vi "Scan Engine-Single Frame.vi"(8 "Error in":errorcluster, 10 "Scan Status":enum16{"Start", "Continue Scan", "Finish Scan"}(ring)=enum."Continue Scan", 11 "Scan Type in":T1) -> (0 "Error Out":errorcluster, 3 "data out":sgl[](array[numeric]))   [LabVIEW 2018]
uses:
  Controls/ScanType.ctl
  Hardware Mfg/AlazarTech SDK/Controls/Alazar Engine Actions.ctl
  Controls/Queue Manager Actions.ctl
  Controls/FGV Actions.ctl
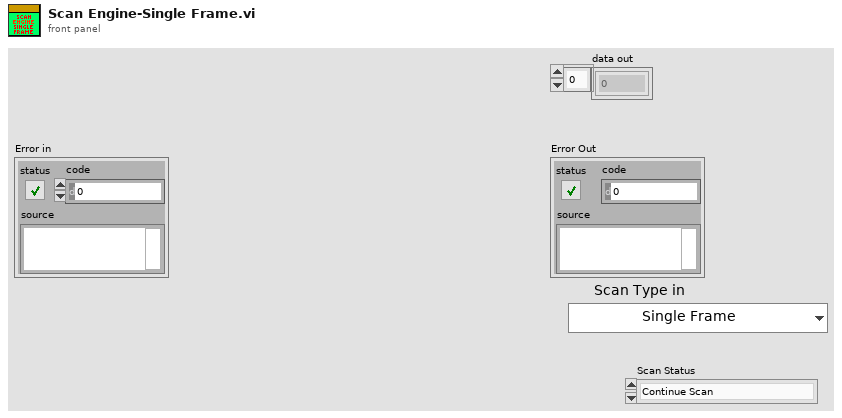
[diagram p1: front panel]
types:
  T1 = typedef "ScanType.ctl" = enum16{"Single Frame", "Continuous Frame", "ROI Line", "Vibratome", "Mosaic", "Mosaic + Slice"}
  T2 = typedef "FGV Actions.ctl" = enum16{"Init", "Set", "Get", "Clear"}
  T3 = typedef "Alazar Engine Actions.ctl" = enum16{"Init", "Config Clock", "Config Ch", "Config Trig", "Config Non-FFT Acq.", "Non-FFT Acquire", "Load background from Non-FFT buffer", "enable background subtrac", "disable background subtrac", "load background from file", "load background from elsewhere", "start acquire", "background subtraction", "Config Acq.", "Acquire", "UnInit"}
  T4 = enum16{"Configure channels", "Write Scan Pattern", "Start Galvo Task", "Is Task Done?", "Stop Galvo", "Uninit", "Init: Calc scan pattern"}
  T5 = typedef "Queue Manager Actions.ctl" = enum16{"Init", "Enqueue", "Enqueue All", "Preview Queue", "Dequeue", "Get Status", "Flush Queue", "Flush All Queues", "Release All Queues", "Release Queue", "Enqueue at Opposite End"}
  T6 = typedef "Alazar parameters.ctl" = cluster{"Trigger Settings":cluster{"General Trigger Settings":T7, "Trigger Engine 1":T8, "Trigger Engine 2":T8}, "Capture Clock":T9, "Device ID":T10, "Ch A Input Control":T11, "Ch B Input Control":T11, "Acq Settings":T12, "Cluster":T13}
  T7 = typedef "General Trigger Settings.ctl" = cluster{"Trigger Operation":u32, "Coupling ID":u32, "Range ID":u32, "Delay":u32, "Timeout Ticks":u32, "Mode":u32, "Parameter":u32}
  T8 = typedef "Trigger Engine Controls.ctl" = cluster{"Trigger Engine":u32, "Source":u32, "Slope":u32, "Level":u32}
  T9 = typedef "Clock Controls.ctl" = cluster{"Sample Rate":u32, "Decimation":u32, "Source":u32, "Edge":u32}
  T10 = typedef "Alazar Device ID.ctl" = cluster{"System ID":u32, "Board ID":u32}
  T11 = typedef "Channel Input Controls.ctl" = cluster{"Channel":u8, "Coupling":u32, "Range":u32, "Impedance":u32}
  T12 = typedef "Alazar Acquisition Settings.ctl" = cluster{"Window Type":u32, "Record Length":u32, "Footer":u32, "Output Format":u32, "Offset":u32, "Records Per Buffer":u32, "Samples per record":u32, "Records Count (Records/Acq)":u32}
  T13 = typedef "Control cluster.ctl" = cluster{"FFT value magnification":dbl, "max queue size (-1, unlimited)":i32, "File Type":T14, "file path":path, "#A-lines to save":u32, "#Z pixels to save":u32, "ImageDescription":string, "Convert to U16?":bool}
  T14 = typedef "file type.ctl" = enum16{"text", "Tiff", "binary"}
  T15 = cluster{"General Trigger Settings":T7, "Trigger Engine 1":T8, "Trigger Engine 2":T8}
  T16 = typedef "Galvo parameters.ctl" = cluster{"Galvo HW Parameters":cluster{"Analog Out Channel":tag, "Min Voltage":dbl, "Max Voltage":dbl, "Pixel Clock Source":tag, "Sample Rate":dbl, "Line Clock Out Ch":tag}, "System Parameters":T17}
  T17 = typedef "System Parameters.ctl" = cluster{"Optical Parameters":T18, "Vibratome":T19, "Table Stages":T20, "Imaging Parameter":T23}
  T18 = typedef "Optical Parameters.ctl" = cluster{"Obj. Focal Length [mm]":dbl, "Scan Lens EFL[mm]":dbl, "Tube Lens EFL[mm]":dbl, "Galvo V Range (+/-)":dbl, "Galvo Max Half Angle [Deg]":dbl, "Max Galvo Range[%]":dbl}
  T19 = typedef "Vibratome Parameters.ctl" = cluster{"Z Bottom [mm]":dbl, "Pre Cut Dwell [s]":dbl, "Blade Frequency [RPM]":u16, "Slice Speed [mm/s]":dbl, "Post Cut Dwell [s]":dbl, "Ramp Time [s]":dbl, "Start X [mm]":dbl, "Start Y [mm]":dbl, "Slice Length [mm]":dbl, "Slice Axis":enum16{"X Axis", "Y Axis", "Z Axis"}, "Controller VISA Ref":refnum<visa-resource-name>}
  T20 = typedef "Translation Stage Parameters.ctl" = cluster{"X Stage":T21, "Y Stage":T21, "Z Stage":T21}
  T21 = typedef "Translation Stage Cluster.ctl" = cluster{"Position":dbl, "Is.Enabled?":bool, "Is.Connected?":bool, "Device SN":string, "AccelerationMaximum":dbl, "VelocityMaximum":dbl, "Acceleration":dbl, "Velocity":dbl, "waitTimeout (ms)":i32, "Model":T22, "Is.Homed?":bool}
  T22 = typedef "Translation Stage Types.ctl" = enum16{"None", "Thorlabs LTS", "Thorlabs MLJ"}
  T23 = typedef "Imaging Parameters.ctl" = cluster{"Raster Scan Direction":T24, "Pixel Dwell Time [Clock Cycles]":u16, "Flyback Time [Clock Cycles]":u16, "XY Center [um]":cluster{"X":dbl, "Y":dbl}, "Pixel Step Size [um]":dbl, "XY Image Size":enum16{"32 x 32", "64 x 64", "128 x 128", "256 x 256", "512 x 512", "1024 x 1024", "2048 x 2048"}, "Custom":bool, "Custom Size":cluster{"X":u16, "Y":u16}, "Line Averages":u8}
  T24 = typedef "Scan Direction.ctl" = enum16{"Uni Directional", "Bi Directional", "None"}
  T25 = cluster{"Analog Out Channel":tag, "Min Voltage":dbl, "Max Voltage":dbl, "Pixel Clock Source":tag, "Sample Rate":dbl, "Line Clock Out Ch":tag}
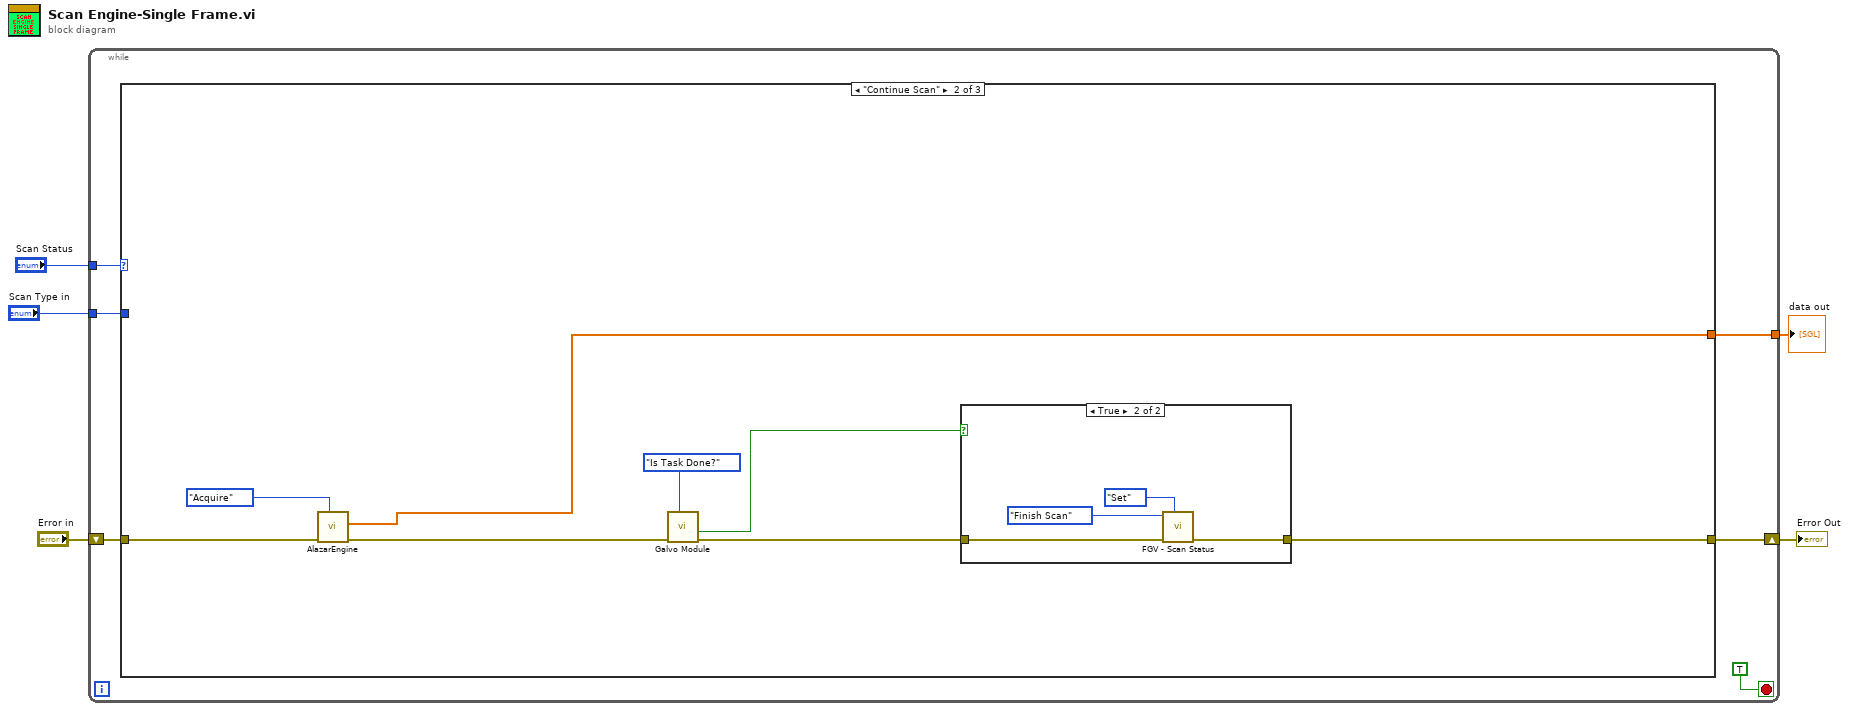
[diagram p0: block diagram]
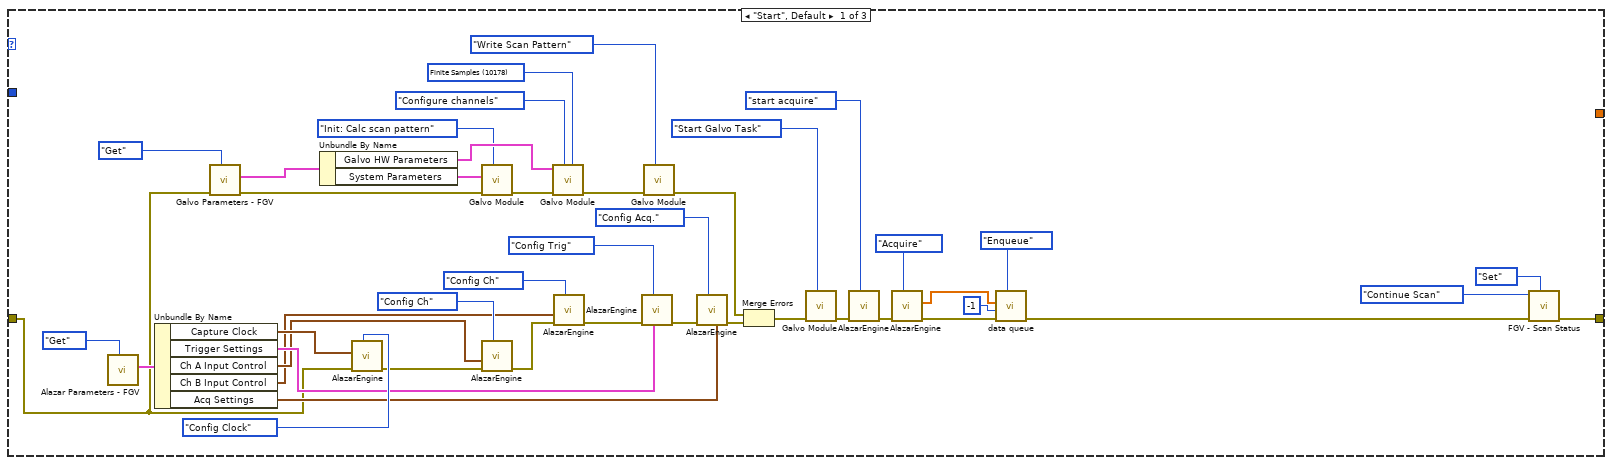
[diagram p2: hidden frame]
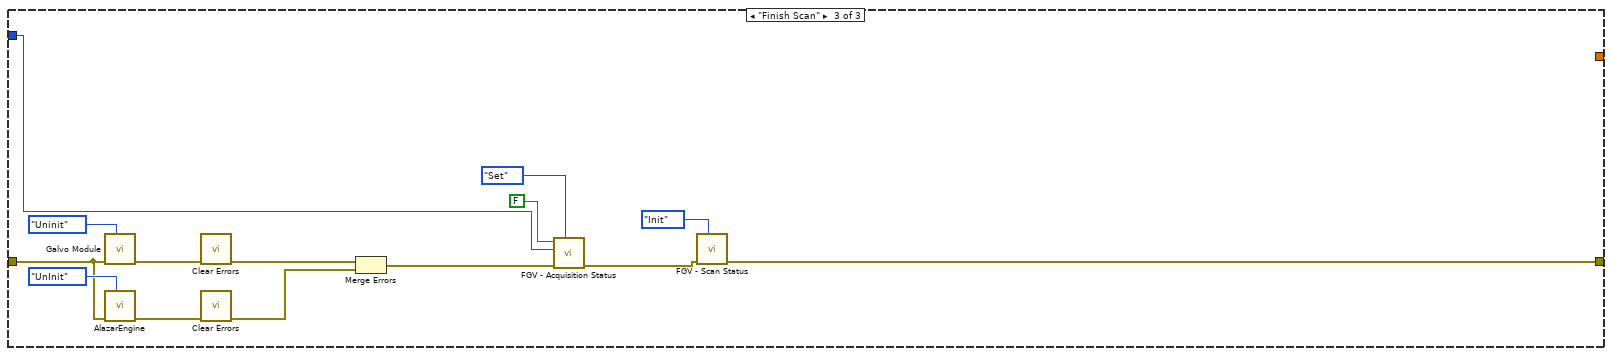
[diagram p4: hidden frame]
diagram:
  n1 = while {
    shift-right: [w10] -> w4
    shift-left: "Error in" -> [w7]
    tunnel: "Scan Type in" -> [w9]
    tunnel: "Scan Status" -> [w8]
    tunnel: [w6] -> w1
    stop <- TRUE ("Status In") stop-if-true
    n2 = case shown="\"Continue Scan\"" w8 {
      tunnel: w7 -> [w16 w61 w78]
      tunnel: [w15 w60 w69] -> w10
      tunnel: w9 -> [_ _ w72]
      tunnel: [_ w56 _] -> w6
      frame "Start", Default {
        w42 = 10178 items=["Finite Samples"=10178, "Continuous Samples"=10123, "Hardware Timed Single Point"=12522] ("sample mode")
        n3 = call "Alazar Parameters - FGV.vi"("Actions"=FGV_Actions."Get") -> ("Alazar parameters out"=w28:T6)  [unwired: 9 in, 1 out]
        n4 = Unbundle By Name(w28) -> ("Capture Clock"=w27:T9, "Trigger Settings"=w26:T15, "Ch A Input Control"=w25:T11, "Ch B Input Control"=w24:T11, "Acq Settings"=w23:T12)
        n5 = call "Galvo Parameters - FGV.vi"("Actions"=FGV_Actions."Get", "Error In"=w16) -> ("Error Out"=w49:errorcluster, "Galvo parameters out"=w44:T16)  [unwired: 8 in]
        n6 = Unbundle By Name(w44) -> ("Galvo HW Parameters"=w47:T25, "System Parameters"=w48:T17)
        n7 = call "AlazarEngine.vi"("Action"=Alazar_Engine_Actions."Config Clock", "error in (no error)"=w16, "Capture Clock"=w27) -> ("error out"=w31:errorcluster)  [unwired: 7 in, 1 out]
        n8 = call "Galvo Module.vi"("Action"=T4."Init: Calc scan pattern", "error in (no error)"=w49, "System Parameters"=w48) -> ("error out"=w45:errorcluster)  [unwired: 7 in, 1 out]
        n9 = call "AlazarEngine.vi"("Action"=Alazar_Engine_Actions."Config Ch", "error in (no error)"=w31, "Ch Input Control"=w25) -> ("error out"=w38:errorcluster)  [unwired: 7 in, 1 out]
        n10 = call "Galvo Module.vi"("sample mode"=w42, "Action"=T4."Configure channels", "error in (no error)"=w45, "Galvo HW Parameters"=w47) -> ("error out"=w46:errorcluster)  [unwired: 6 in, 1 out]
        n11 = call "AlazarEngine.vi"("Action"=Alazar_Engine_Actions."Config Ch", "error in (no error)"=w38, "Ch Input Control"=w24) -> ("error out"=w35:errorcluster)  [unwired: 7 in, 1 out]
        n12 = call "AlazarEngine.vi"("Trigger Settings"=w26, "Action"=Alazar_Engine_Actions."Config Trig", "error in (no error)"=w35) -> ("error out"=w32:errorcluster)  [unwired: 7 in, 1 out]
        n13 = call "Galvo Module.vi"("Action"=T4."Write Scan Pattern", "error in (no error)"=w46) -> ("error out"=w22:errorcluster)  [unwired: 8 in, 1 out]
        n14 = call "AlazarEngine.vi"("Acq Settings"=w23, "Action"=Alazar_Engine_Actions."Config Acq.", "error in (no error)"=w32) -> ("error out"=w21:errorcluster)  [unwired: 7 in, 1 out]
        n15 = Merge Errors(w22, w21) -> (w18:errorcluster)
        n16 = call "Galvo Module.vi"("Action"=T4."Start Galvo Task", "error in (no error)"=w18) -> ("error out"=w17:errorcluster)  [unwired: 8 in, 1 out]
        n17 = call "AlazarEngine.vi"("Action"=Alazar_Engine_Actions."start acquire", "error in (no error)"=w17) -> ("error out"=w55:errorcluster)  [unwired: 8 in, 1 out]
        n18 = call "AlazarEngine.vi"("Action"=Alazar_Engine_Actions."Acquire", "error in (no error)"=w55) -> ("error out"=w51:errorcluster, "Buffer"=w50:sgl[])  [unwired: 8 in]
        n19 = call "data queue.vi"("Action"=Queue_Manager_Actions."Enqueue", "error in (no error)"=w51, "timeout in ms (-1)"=-1, "data in"=w50) -> ("error out"=w12:errorcluster)  [unwired: 4 in, 3 out]
        n20 = call "FGV - Scan Status.vi"("Actions"=FGV_Actions."Set", "Error In"=w12, "Scan Status in"=enum16{"Start", "Continue Scan", "Finish Scan"}."Continue Scan") -> ("Error Out"=w15:errorcluster)  [unwired: 6 in, 2 out]
      }
      frame "Continue Scan" {
        n21 = call "AlazarEngine.vi"("Action"=Alazar_Engine_Actions."Acquire", "error in (no error)"=w61) -> ("error out"=w57:errorcluster, "Buffer"=w56:sgl[])  [unwired: 8 in]
        n22 = call "Galvo Module.vi"("Action"=T4."Is Task Done?", "error in (no error)"=w57) -> ("error out"=w59:errorcluster, "task done?"=w58:bool)  [unwired: 8 in]
        n23 = case shown="True" w58 {
          tunnel: w59 -> [w64 w67]
          tunnel: [w64 w66] -> w60
          frame False {
          }
          frame True {
            n24 = call "FGV - Scan Status.vi"("Actions"=FGV_Actions."Set", "Error In"=w67, "Scan Status in"=enum16{"Start", "Continue Scan", "Finish Scan"}."Finish Scan") -> ("Error Out"=w66:errorcluster)  [unwired: 6 in, 2 out]
          }
        }
      }
      frame "Finish Scan" {
        n25 = call "Galvo Module.vi"("Action"=T4."Uninit", "error in (no error)"=w78) -> ("error out"=w81:errorcluster)  [unwired: 8 in, 1 out]
        n26 = call "AlazarEngine.vi"("Action"=Alazar_Engine_Actions."UnInit", "error in (no error)"=w78) -> ("error out"=w80:errorcluster)  [unwired: 8 in, 1 out]
        n27 = call <vilib>:"Clear Errors.vi"("error in (no error)"=w81) -> ("error out"=w77:errorcluster)  [unwired: 5 in, 1 out]
        n28 = call <vilib>:"Clear Errors.vi"("error in (no error)"=w80) -> ("error out"=w76:errorcluster)  [unwired: 5 in, 1 out]
        n29 = Merge Errors(w77, w76) -> (w73:errorcluster)
        n30 = call "FGV - Acquisition Status.vi"("Actions"=FGV_Actions."Set", "Error In"=w73, "Scan Type [In]"=w72, "Status In"=FALSE) -> ("Error Out"=w70:errorcluster)  [unwired: 5 in, 2 out]
        n31 = call "FGV - Scan Status.vi"("Actions"=FGV_Actions."Init", "Error In"=w70) -> ("Error Out"=w69:errorcluster)  [unwired: 7 in, 2 out]
      }
    }
  }
  "Error Out" <- w4
  "data out" <- w1
